vi "Init.ZMQ.vi"(1 "endpoint":string="tcp://*:10000") -> (0 "socket":refnum<class "zmq_socket.lvclass">)   [LabVIEW 2014]
uses:
  <vilib>/addons/zeromq/zmq_socket.lvclass
  <vilib>/addons/zeromq/socket_type.ctl
  ZMQ.global.vi
  <vilib>/addons/zeromq/zmq_context.lvclass
  <vilib>/addons/zeromq/zeromq.lvlib
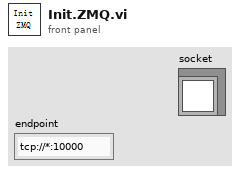
[diagram p1: front panel]
types:
  T1 = cluster{"context":refnum<class "zmq_context.lvclass">, "socket":refnum<class "zmq_socket.lvclass">, "endpoint":string}
  T2 = typedef "zeromq.lvlib/socket_type.ctl" = enum8{"ZMQ_PAIR", "ZMQ_PUB", "ZMQ_SUB", "ZMQ_REQ", "ZMQ_REP", "ZMQ_DEALER", "ZMQ_ROUTER", "ZMQ_PULL", "ZMQ_PUSH", "ZMQ_XPUB", "ZMQ_XSUB"}
  T3 = cluster{"context out":refnum<class "zmq_context.lvclass">, "socket out":refnum<class "zmq_socket.lvclass">, "endpoint":string}
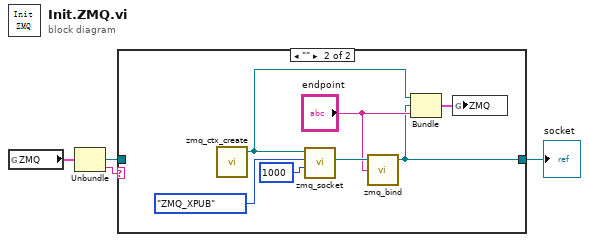
[diagram p0: block diagram]
diagram:
  n1 = global read "ZMQ.global.vi" "ZMQ"() -> (w3:T1)
  n2 = Unbundle(w3) -> ("socket"=w1:refnum<class "zmq_socket.lvclass">, "endpoint"=w4:string)  [unwired: 1 out]
  n3 = case shown="\"\"" w4 {
    tunnel: [w5 w7] -> w2
    tunnel: w1 -> [w5 _]
    frame Default {
    }
    frame "" {
      n4 = call <vilib>:"zmq_ctx_create.vi"() -> ("context out"=w9:refnum<class "zmq_context.lvclass">)  [unwired: 4 in, 1 out]
      n5 = call <vilib>:"zmq_socket.vi"("linger (ms)"=1000, "socket type"=socket_type."ZMQ_XPUB", "context in"=w9) -> ("socket out"=w12:refnum<class "zmq_socket.lvclass">)  [unwired: 2 in, 2 out]
      n6 = call <vilib>:"zmq_bind.vi"("endpoint"="endpoint", "socket in"=w12) -> ("socket out"=w7:refnum<class "zmq_socket.lvclass">)  [unwired: 2 in, 1 out]
      n7 = Bundle("context out"=w9, "socket out"=w7, "endpoint"="endpoint") -> (w6:T3)  [unwired: 1 in]
      n8 = global write "ZMQ.global.vi" "ZMQ"(w6) -> ()
    }
  }
  "socket" <- w2
